vi "Defer Panel Updates.vi"(8 "error in (no error)":errorcluster, 10 "Refnums for FP Objects":T5, 11 "State in":T1={"Graph Visible Items"={"Plot Legend"=FALSE, "Scale Legend"=FALSE, "Graph Palette"=FALSE, "Cursor Legend"=FALSE, "X Scrollbar"=FALSE}, "View Table"=FALSE, "Table Visible Items"={"Vertical Scrollbar"=FALSE, "Horizontal Scrollbar"=FALSE, "Row Headers"=FALSE, "Column Headers"=FALSE, "Vertical Lines"=FALSE, "Horizontal Lines"=FALSE}, "Header Font"={"Font Name"="", "Size"=0, "Bold"=FALSE, "Italic"=FALSE, "Underline"=FALSE, "Strikeout"=FALSE, "Color"=0}, "Cell Font"={"Font Name"="", "Size"=0, "Bold"=FALSE, "Italic"=FALSE, "Underline"=FALSE, "Strikeout"=FALSE, "Color"=0}, "Description and Tip..."={"Description"="", "Tip"=""}, "Moveable Splitter Position"=0, "Measurement Cursor Configuration"={"XY"={"enable XY"=FALSE, "Position (X)"=[], "Type"=enum."Absolute", "Y reference"=0.0, "color"=0}, "band"={"enable band"=FALSE, "B1"=0.0, "B2"=0.0, "Fixed bandwidth (B2-B1)"=0.0, "B1 color"=0, "B2 color"=0}, "harmonic"={"enable harmonics"=FALSE, "X reference (1X)"=0.0, "Maximum"=0, "Subset"=enum."All", "1X color"=0, "MX color"=0}, "sideband"={"enable sideband"=FALSE, "X center (C)"=0.0, "Sidebands"=0, "X spacing (s)"=0.0, "Center color"=0, "Sideband color"=0}}, "Cursors"={"List"=[], "Tags"=[]}, "X Increment"=0.0, "X Scale"={"Label Visible"=FALSE, "Label Text"="", "Mapping Mode"=0, "Format String"=""}, "Y Scale"={"Label Visible"=FALSE, "Label Text"="", "Mapping Mode"=0, "Format String"=""}, "Colors"={"background"=16777215, "major grid"=8355711, "minor grid"=12632256, "font"=0}, "desired spectrum view"={"scaling"={"linear/dB"=enum."no change", "dB reference"=0.0, "power/magnitude"=enum."no change", "view"=enum."no change"}, "spectral density"=enum."no change"}, "Plot Color Wheel"=[3381759, 32768, 982784, 4375295, 13827953, 13457919, 16757522, 4343295, 16728758, 12095254], "Plots"=[], "registered user events"=variant, "Lock 1X to Peak"=FALSE, "spectrum component"=32, "phase spectrum view"={"desired units"=0, "desired wrapping"=4}} caption="State" {"phase spectrum view"."desired wrapping" items=["No change", "Unwrap", "Wrap: -360 to 0", "Wrap: -270 to 90", "Wrap: -180 to 180", "Wrap: -90 to 270", "Wrap: 0 to 360", "Wrap: custom range"]; "phase spectrum view"."desired units" items=["No change", "Radians", "Degrees", "Cycles"]; "spectrum component" items=["Magnitude^2"=37, "Magnitude"=32, "Phase"=33, "Real"=34, "Imaginary"=35, "Coherence"=36, "Unknown"=99]; "Y Scale"."Mapping Mode" items=["Linear", "Logarithmic"]; "X Scale"."Mapping Mode" items=["Linear", "Logarithmic"]}) -> (0 "error out":errorcluster, 3 "State out":T1={"Graph Visible Items"={"Plot Legend"=FALSE, "Scale Legend"=FALSE, "Graph Palette"=FALSE, "Cursor Legend"=FALSE, "X Scrollbar"=FALSE}, "View Table"=FALSE, "Table Visible Items"={"Vertical Scrollbar"=FALSE, "Horizontal Scrollbar"=FALSE, "Row Headers"=FALSE, "Column Headers"=FALSE, "Vertical Lines"=FALSE, "Horizontal Lines"=FALSE}, "Header Font"={"Font Name"="", "Size"=0, "Bold"=FALSE, "Italic"=FALSE, "Underline"=FALSE, "Strikeout"=FALSE, "Color"=0}, "Cell Font"={"Font Name"="", "Size"=0, "Bold"=FALSE, "Italic"=FALSE, "Underline"=FALSE, "Strikeout"=FALSE, "Color"=0}, "Description and Tip..."={"Description"="", "Tip"=""}, "Moveable Splitter Position"=0, "Measurement Cursor Configuration"={"XY"={"enable XY"=FALSE, "Position (X)"=[], "Type"=enum."Absolute", "Y reference"=0.0, "color"=0}, "band"={"enable band"=FALSE, "B1"=0.0, "B2"=0.0, "Fixed bandwidth (B2-B1)"=0.0, "B1 color"=0, "B2 color"=0}, "harmonic"={"enable harmonics"=FALSE, "X reference (1X)"=0.0, "Maximum"=0, "Subset"=enum."All", "1X color"=0, "MX color"=0}, "sideband"={"enable sideband"=FALSE, "X center (C)"=0.0, "Sidebands"=0, "X spacing (s)"=0.0, "Center color"=0, "Sideband color"=0}}, "Cursors"={"List"=[], "Tags"=[]}, "X Increment"=0.0, "X Scale"={"Label Visible"=FALSE, "Label Text"="", "Mapping Mode"=0, "Format String"=""}, "Y Scale"={"Label Visible"=FALSE, "Label Text"="", "Mapping Mode"=0, "Format String"=""}, "Colors"={"background"=16777215, "major grid"=8355711, "minor grid"=12632256, "font"=0}, "desired spectrum view"={"scaling"={"linear/dB"=enum."no change", "dB reference"=0.0, "power/magnitude"=enum."no change", "view"=enum."no change"}, "spectral density"=enum."no change"}, "Plot Color Wheel"=[3381759, 32768, 982784, 4375295, 13827953, 13457919, 16757522, 4343295, 16728758, 12095254], "Plots"=[], "registered user events"=variant, "Lock 1X to Peak"=FALSE, "spectrum component"=32, "phase spectrum view"={"desired units"=0, "desired wrapping"=4}} caption="State" {"phase spectrum view"."desired wrapping" items=["No change", "Unwrap", "Wrap: -360 to 0", "Wrap: -270 to 90", "Wrap: -180 to 180", "Wrap: -90 to 270", "Wrap: 0 to 360", "Wrap: custom range"]; "phase spectrum view"."desired units" items=["No change", "Radians", "Degrees", "Cycles"]; "spectrum component" items=["Magnitude^2"=37, "Magnitude"=32, "Phase"=33, "Real"=34, "Imaginary"=35, "Coherence"=36, "Unknown"=99]; "Y Scale"."Mapping Mode" items=["Linear", "Logarithmic"]; "X Scale"."Mapping Mode" items=["Linear", "Logarithmic"]})   [LabVIEW 2017, in "Spectrum with Cursors.xctl"]
uses:
  <vilib>/addons/_XControls/Spectrum with Cursors/Spectrum with Cursors.xctl
  <vilib>/addons/_XControls/Spectrum with Cursors/Controls/Refnums Typedef.ctl
  <vilib>/addons/_XControls/Spectrum with Cursors/Controls/State.ctl
  <vilib>/Utility/miscctls.llb/LVFontTypeDef.ctl
  <vilib>/addons/_XControls/Spectrum with Cursors/Controls/Measurement Cursor Configuration.ctl
  <vilib>/addons/_NISVFA/_Shared subVIs/Controls/NI Spectrum Component.ctl
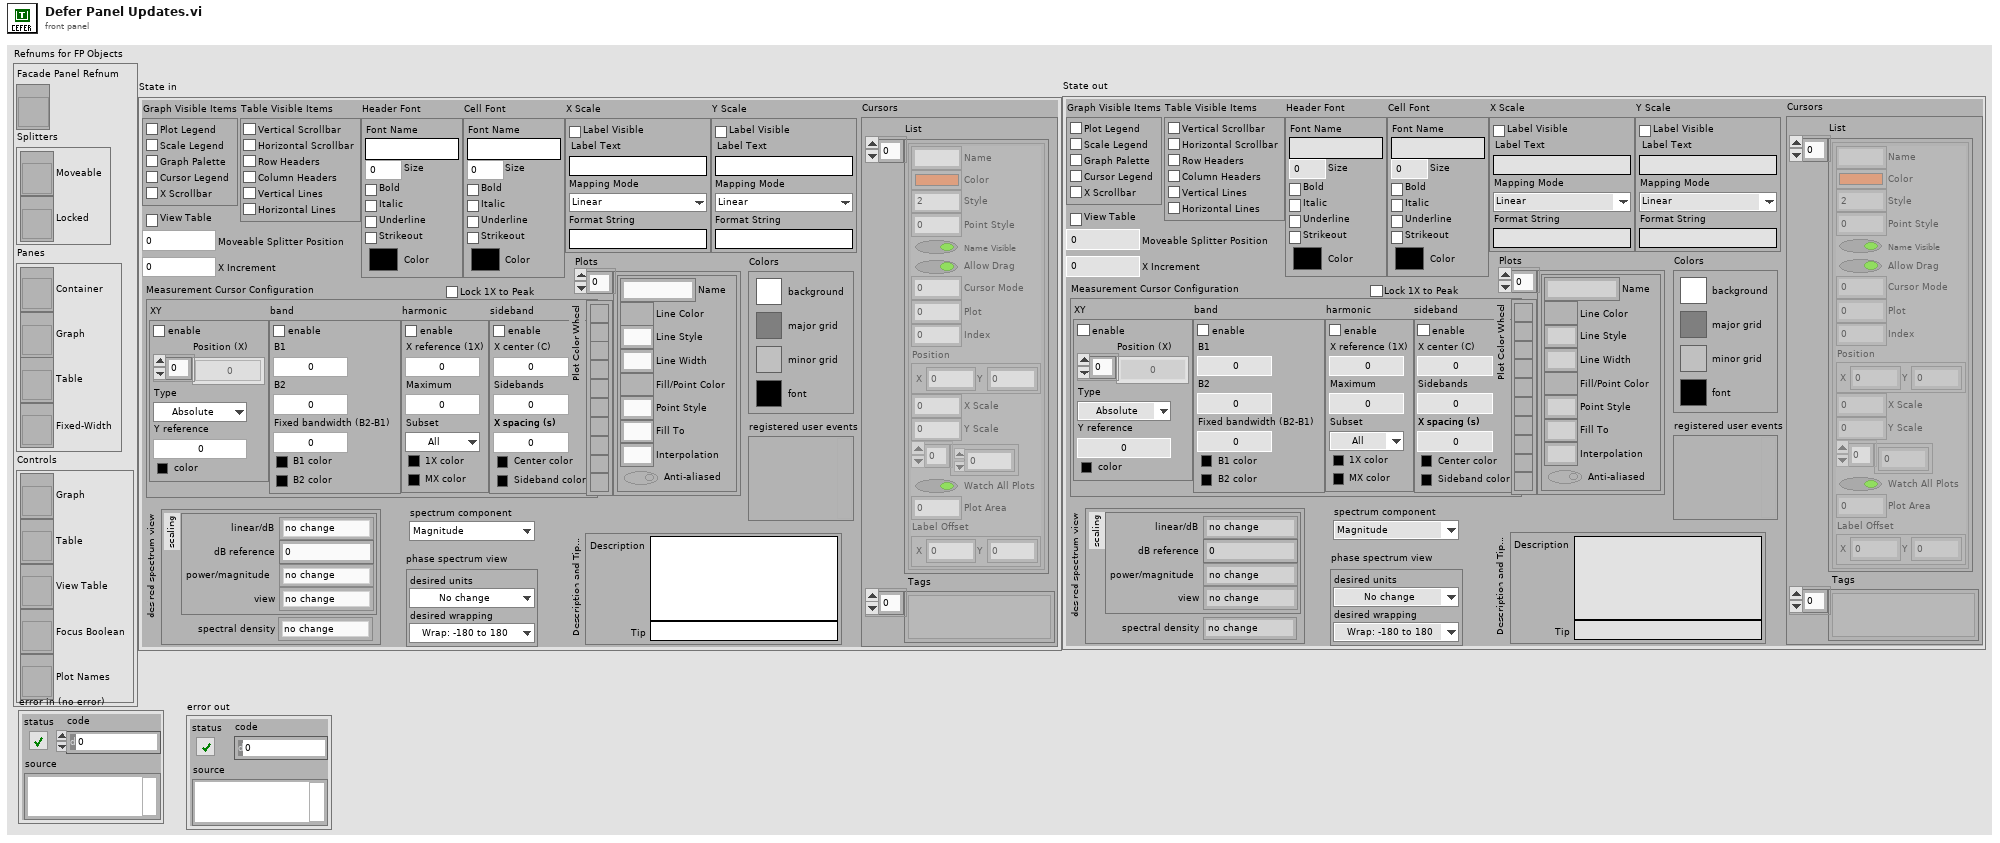
[diagram p1: front panel]
types:
  T1 = typedef "Spectrum with Cursors.xctl/State.ctl" = cluster{"Graph Visible Items":cluster{"Plot Legend":bool, "Scale Legend":bool, "Graph Palette":bool, "Cursor Legend":bool, "X Scrollbar":bool}, "View Table":bool, "Table Visible Items":cluster{"Vertical Scrollbar":bool, "Horizontal Scrollbar":bool, "Row Headers":bool, "Column Headers":bool, "Vertical Lines":bool, "Horizontal Lines":bool}, "Header Font":T2, "Cell Font":T2, "Description and Tip...":cluster{"Description":string, "Tip":string}, "Moveable Splitter Position":i32, "Measurement Cursor Configuration":T3, "Cursors":cluster{"List":cluster{"Name":string, "Color":u32, "Style":i32, "Point Style":u8, "Name Visible":bool, "Allow Drag":bool, "Cursor Mode":u32, "Plot":i32, "Index":i32, "Position":cluster{"X":dbl, "Y":dbl}, "X Scale":u32, "Y Scale":u32, "Watch Plots":i32[], "Watch All Plots":bool, "Plot Area":i32, "Label Offset":cluster{"X":dbl, "Y":dbl}}[], "Tags":variant[]}, "X Increment":dbl, "X Scale":cluster{"Label Visible":bool, "Label Text":string, "Mapping Mode":u8, "Format String":string}, "Y Scale":cluster{"Label Visible":bool, "Label Text":string, "Mapping Mode":u8, "Format String":string}, "Colors":cluster{"background":u32, "major grid":u32, "minor grid":u32, "font":u32}, "desired spectrum view":cluster{"scaling":cluster{"linear/dB":enum16{"no change", "linear", "dB"}, "dB reference":dbl, "power/magnitude":enum16{"no change", "power", "magnitude"}, "view":enum16{"no change", "rms", "peak", "peak-peak"}}, "spectral density":enum16{"no change", "spectrum", "spectral density"}}, "Plot Color Wheel":u32[], "Plots":cluster{"Name":string, "Line Color":u32, "Line Style":u8, "Line Width":u8, "Fill/Point Color":u32, "Point Style":u8, "Fill To":i16, "Interpolation":u8, "Anti-aliased":bool}[], "registered user events":variant, "Lock 1X to Peak":bool, "spectrum component":T4, "phase spectrum view":cluster{"desired units":u16, "desired wrapping":u16}}
  T2 = typedef "LVFontTypeDef.ctl" = cluster{"Font Name":string, "Size":u16, "Bold":bool, "Italic":bool, "Underline":bool, "Strikeout":bool, "Color":u32}
  T3 = typedef "Spectrum with Cursors.xctl/Measurement Cursor Configuration.ctl" = cluster{"XY":cluster{"enable XY":bool, "Position (X)":dbl[], "Type":enum16{"Absolute", "Relative"}, "Y reference":dbl, "color":u32}, "band":cluster{"enable band":bool, "B1":dbl, "B2":dbl, "Fixed bandwidth (B2-B1)":dbl, "B1 color":u32, "B2 color":u32}, "harmonic":cluster{"enable harmonics":bool, "X reference (1X)":dbl, "Maximum":i32, "Subset":enum16{"All", "Even", "Odd"}, "1X color":u32, "MX color":u32}, "sideband":cluster{"enable sideband":bool, "X center (C)":dbl, "Sidebands":i32, "X spacing (s)":dbl, "Center color":u32, "Sideband color":u32}}
  T4 = typedef "NI Spectrum Component.ctl" = u16
  T5 = typedef "Spectrum with Cursors.xctl/Refnums Typedef.ctl" = cluster{"Facade Panel Refnum":refnum<vi>, "Splitters":cluster{"Moveable":refnum<vi>, "Locked":refnum<vi>}, "Panes":cluster{"Container":refnum<vi>, "Graph":refnum<vi>, "Table":refnum<vi>, "Fixed-Width":refnum<vi>}, "Controls":cluster{"Graph":refnum<vi>, "Table":refnum<vi>, "View Table":refnum<vi>, "Focus Boolean":refnum<vi>, "Plot Names":refnum<vi>}}
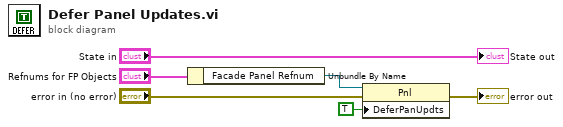
[diagram p0: block diagram]
diagram:
  n1 = Unbundle By Name("Refnums for FP Objects") -> ("Facade Panel Refnum"=w2:refnum<vi>)
  n2 = property class="Pnl"(reference=w2, error in="error in (no error)", "DeferPanUpdts"=TRUE ("Defer Panel Updates")) -> (error out=→"error out":errorcluster)  [unwired: 1 out]
  "State out" <- "State in"
